vi "timing and stabilization test.vi"() -> ()   [LabVIEW 2013, in "Timing and Stabilization.lvlib"]
uses:
  Timing and Stabilization.lvlib
  Stabilization.ctl
  MeasurementControl Message Queue Folder/MeasurementControl Message Queue.lvlib
panel:
  out "Stabilization Data":T1={"Stabilization waveform"={"t0"=timestamp(0 s since 1904-01-01), "dt"=50.0, "Y"=[10.0, 9.0, 8.75, 8.5, 8.25, 8.125, 8.06, 8.03, 8.015, 8.0, 8.0, 8.0]}, "Variation"=0.0, "Stabilized"=FALSE, "Threshold"=0.0, "time to stabilize"=0.0, "3 points"=[]}
  in  "Start Insulated Sphere Timer":bool
  in  "Reset Insulated Sphere Timer":bool
  in  "Start Naked Sphere Timer":bool
  out "Message":string
  in  "Reset Naked Sphere Timer":bool
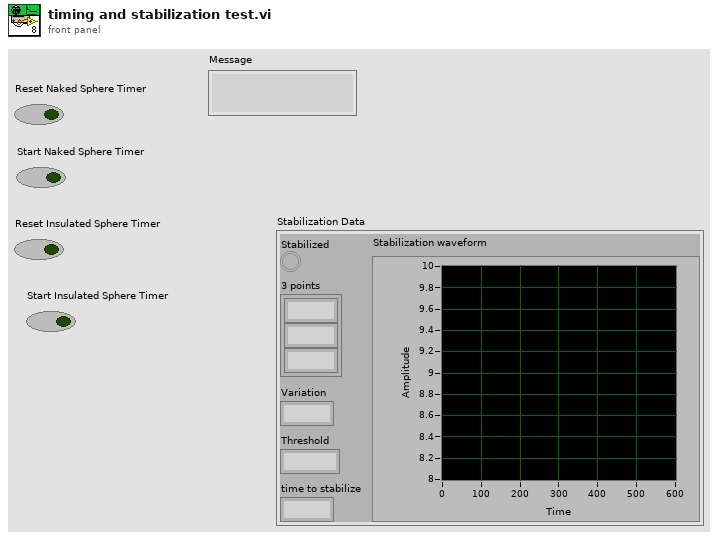
[diagram p1: front panel]
types:
  T1 = typedef "Timing and Stabilization.lvlib/Stabilization.ctl" = cluster{"Stabilization waveform":waveform(dbl), "Variation":dbl, "Stabilized":bool, "Threshold":dbl, "time to stabilize":dbl, "3 points":dbl[]}
  T2 = typedef "MeasurementControl Message Queue.lvlib/All Message Queues.ctl" = cluster{"Master":refnum<queue>, "UI":refnum<queue>, "Stabilization":refnum<queue>, "Logging":refnum<queue>, "Timing":refnum<queue>}
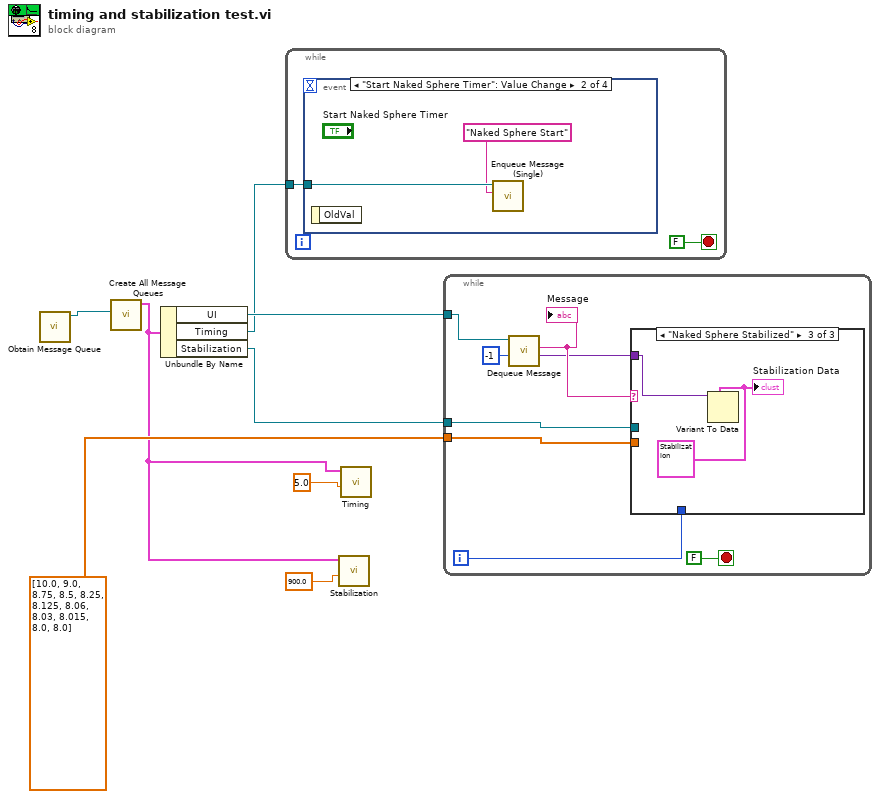
[diagram p0: block diagram]
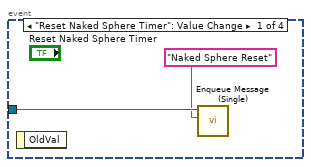
[diagram p2: hidden frame]
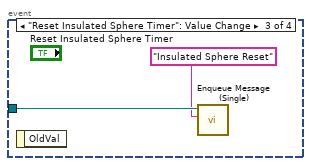
[diagram p3: hidden frame]
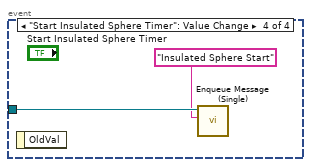
[diagram p4: hidden frame]
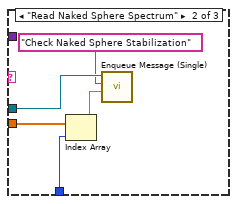
[diagram p6: hidden frame]
diagram:
  n1 = call "Obtain Message Queue.vi"() -> ("Message Queue"=w8:refnum<queue>)  [unwired: 10 in, 1 out]
  n2 = call "Create All Message Queues.vi"("Master Queue In"=w8) -> ("Message Queues out"=w1:T2)  [unwired: 9 in, 1 out]
  n3 = Unbundle By Name(w1) -> ("UI"=w7:refnum<queue>, "Timing"=w3:refnum<queue>, "Stabilization"=w5:refnum<queue>)
  n4 = while {
    tunnel: w3 -> [w10]
    stop <- FALSE stop-if-true
    n5 = event shown="[1] \"Start Naked Sphere Timer\": Value Change" {
      selector: _ -> [_ _ _ _]
      dyn-events: _ -> [_ _ _ _]
      timeout: _ -> [_ _ _ _]
      tunnel: w10 -> [w12 w14 w16 w18]
      event "Reset Naked Sphere Timer": Value Change {
        n6 = event-data() -> ()  [unwired: 1 in, 1 out]
        n7 = call "Enqueue Message (Single).vi"("Message"="Naked Sphere Reset", "Message Queue"=w12) -> ()  [unwired: 8 in, 2 out]
      }
      event "Start Naked Sphere Timer": Value Change {
        n8 = event-data() -> ()  [unwired: 1 in, 1 out]
        n9 = call "Enqueue Message (Single).vi"("Message"="Naked Sphere Start", "Message Queue"=w14) -> ()  [unwired: 8 in, 2 out]
      }
      event "Reset Insulated Sphere Timer": Value Change {
        n10 = event-data() -> ()  [unwired: 1 in, 1 out]
        n11 = call "Enqueue Message (Single).vi"("Message"="Insulated Sphere Reset", "Message Queue"=w16) -> ()  [unwired: 8 in, 2 out]
      }
      event "Start Insulated Sphere Timer": Value Change {
        n12 = event-data() -> ()  [unwired: 1 in, 1 out]
        n13 = call "Enqueue Message (Single).vi"("Message"="Insulated Sphere Start", "Message Queue"=w18) -> ()  [unwired: 8 in, 2 out]
      }
    }
  }
  n14 = call "Stabilization.vi"("Stabilization\nInterval"=900.0 ("Stabilization\nInterval"), "Message Queues out"=w1) -> ()  [unwired: 9 in, 1 out]
  n15 = call "Timing.vi"("Stabilization\nInterval"=5.0 ("Stabilization\nInterval"), "Message Queues out"=w1) -> ()  [unwired: 9 in, 1 out]
  n16 = while {
    tunnel: w7 -> [w26]
    tunnel: w5 -> [w22]
    tunnel: dbl[] [10.0, 9.0, 8.75, 8.5, 8.25, 8.125, 8.06, 8.03, 8.015, 8.0, 8.0] -> [w20]
    i -> [w21]
    stop <- FALSE stop-if-true
    n17 = call "Dequeue Message.vi"("timeout in ms (-1)"=-1, "Message Queue"=w26) -> ("Message Data"=w19:variant, "Message"=w23:string)  [unwired: 6 in, 2 out]
    "Message" <- w23
    n18 = case shown="\"Naked Sphere Stabilized\"" w23 {
      tunnel: w22 -> [_ w31 _]
      tunnel: w21 -> [_ w29 _]
      tunnel: w20 -> [_ w28 _]
      tunnel: w19 -> [_ _ w33]
      frame "False", Default {
      }
      frame "Read Naked Sphere Spectrum" {
        n19 = Index Array(array=w28, index=w29) -> (element=w27:dbl)
        n20 = call "Enqueue Message (Single).vi"("Message Data"=w27, "Message"="Check Naked Sphere Stabilization", "Message Queue"=w31) -> ()  [unwired: 7 in, 2 out]
      }
      frame "Naked Sphere Stabilized" {
        w32 = T1 {"Stabilization waveform"={"t0"=timestamp(0 s since 1904-01-01), "dt"=50.0, "Y"=[10.0, 9.0, 8.75, 8.5, 8.25, 8.125, 8.06, 8.03, 8.015, 8.0, 8.0, 8.0]}, "Variation"=0.0, "Stabilized"=FALSE, "Threshold"=0.0, "time to stabilize"=0.0, "3 points"=[]} ("Stabilization Data")
        n21 = Variant To Data(type=w32, Variant=w33) -> ()  [unwired: 1 in, 2 out]
        "Stabilization Data" <- w32
      }
    }
  }
